vi "Read_Sub_Collection.vi"(8 "error in (no error)":errorcluster caption="entrée d'erreur (pas d'erreur)", 11 "Firebase PCBA en entrée":refnum<class "Firebase Benches_Number.lvclass">) -> (0 "error out":errorcluster caption="sortie d'erreur", 2 "Data_Test":T1(array[cluster]), 3 "Firebase PCBA en sortie":refnum<class "Firebase Benches_Number.lvclass">)   [LabVIEW 2020, in "Library Instrument & Equipement.lvlib" / "Library FireBase.lvlib" / "Firebase Benches_Number.lvclass"]
doc: "Return the documents present in the test collection for each DATA read with Get_Data\nPlease initialise the following values\n - Name BDD\n - Document of test sequence\n - API Key\n - Nb To Read"
uses:
  Firebase Benches_Number.lvclass
  Firebase Benches_Number.lvclass/Firebase Benches_Number.ctl
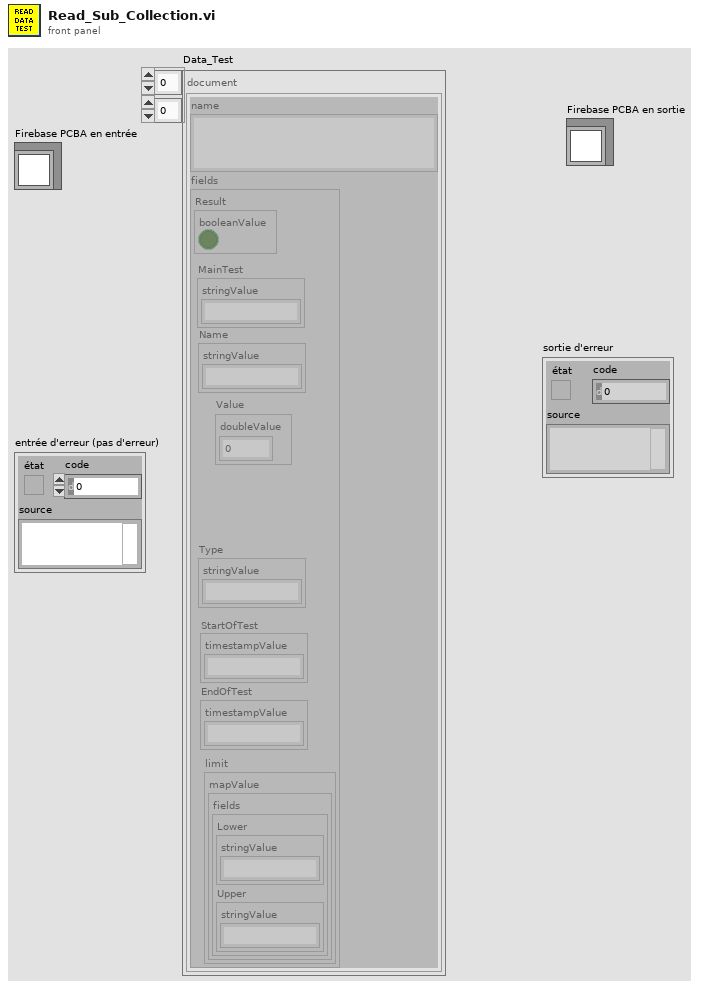
[diagram p1: front panel]
types:
  T1 = cluster{"name":string, "fields":cluster{"Result":cluster{"booleanValue":bool}, "Name":cluster{"stringValue":string}, "StartOfTest":cluster{"timestampValue":string}, "EndOfTest":cluster{"timestampValue":string}, "limit":cluster{"mapValue":cluster{"fields":cluster{"Lower":cluster{"stringValue":string}, "Upper":cluster{"stringValue":string}}}}, "Value":cluster{"doubleValue":dbl}, "Type":cluster{"stringValue":string}, "MainTest":cluster{"stringValue":string}}}[][]
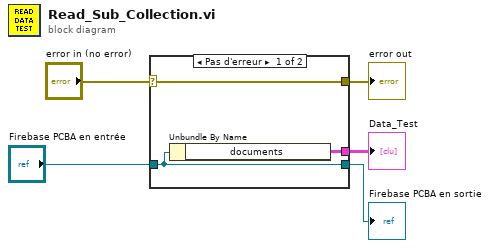
[diagram p0: block diagram]
diagram:
  n1 = case shown="Pas d'erreur" "error in (no error)" {
    selector: "error in (no error)" -> [w7 w10]
    tunnel: [w7 w10] -> w3
    tunnel: [w8 w9] -> w4
    tunnel: "Firebase PCBA en entrée" -> [w8 w9]
    tunnel: [w6 _] -> w1
    frame No Error {
      n2 = Unbundle By Name(w8) -> ("documents"=w6:T1)
    }
    frame Error {
    }
  }
  "error out" <- w3
  "Firebase PCBA en sortie" <- w4
  "Data_Test" <- w1
